vi "test Import Configuration File (Parallel Use).vi"(8 "error in":errorcluster, 11 "TestCase in":refnum<class "Import.lvclass">) -> (0 "error out":errorcluster, 3 "TestCase out":refnum<class "Import.lvclass">)   [LabVIEW 2020, in "Import.lvclass"]
uses:
  Import.lvclass
  <vilib>/addons/_JKI Toolkits/VI Tester/TestCase.llb/TestCase.lvclass
  Import/ARINC 429 Import.lvlib
  niveristand-custom-device-testing-tools/VeriStandTestUtilities/VeriStandTestUtilities.lvlib
  C:/Program Files (x86)/National Instruments/LabVIEW 2020/vi.lib/addons/_JKI Toolkits/VI Tester/TestCase.llb/TestCase.lvclass
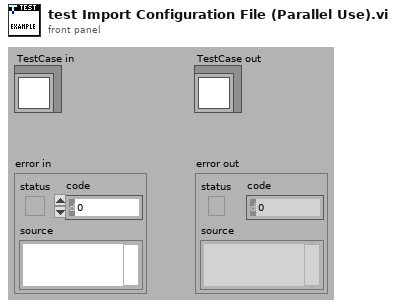
[diagram p1: front panel]
types:
  T1 = typedef "VS Channels Definition for All Labels on Hardware Channel.ctl" = cluster{"hardware channel":i32, "labels":T2[]}
  T2 = typedef "VS Channels Definition for Label.ctl" = cluster{"label (Dec)":u32, "parameters":T3[], "SDI value":u8, "SDI enabled":bool, "transfer type":T7}
  T3 = typedef "VS Channel Definition for Parameter.ctl" = cluster{"name":string, "direction":T4, "default value":dbl, "unit":string, "Parameter":T5}
  T4 = typedef "Direction.ctl" = enum16{"Rx", "Tx"}
  T5 = typedef "Parameter Definition.ctl" = cluster{"start index":i32, "size":i32, "encoding":T6, "signed":bool, "scale multiplier":dbl, "scale offset":dbl}
  T6 = typedef "Encoding and Decoding.lvlib/Encoding.ctl" = enum16{"BNR", "BCD", "Discrete"}
  T7 = typedef "Transfer Type.ctl" = enum16{"Scheduled", "Acyclic", "Block", "Strobe"}
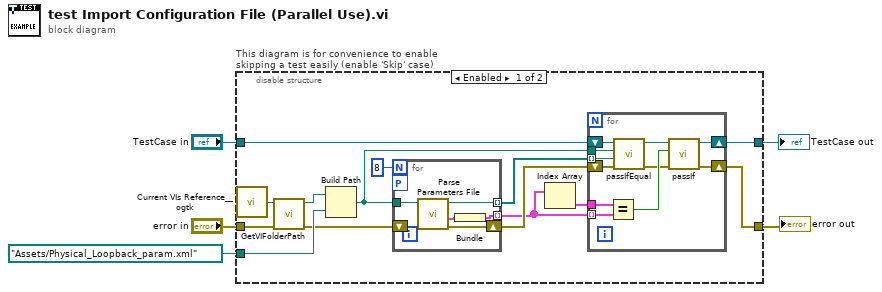
[diagram p0: block diagram]
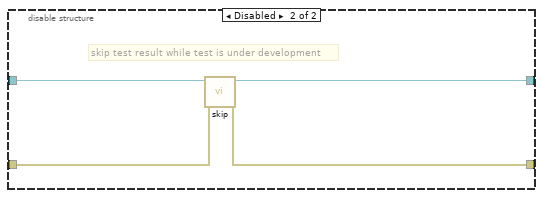
[diagram p2: hidden frame]
diagram:
  n1 = disable-structure "This diagram is for convenience to enable skipping a test easily (enable 'Skip' case)" shown="Enabled" {
    disable-tunnel: "TestCase in" -> [w19 w40]
    disable-tunnel: [w13 w38] -> w2
    disable-tunnel: [w14 w39] -> w4
    disable-tunnel: "error in" -> [w17 w37]
    disable-tunnel: path "Assets/Physical_Loopback_param.xml" ("Absolute or Relative Path") -> [w16 _]
    frame Enabled {
      n2 = call <userlib>:"Current VIs Reference__ogtk.vi"() -> ("Current VI's reference"=w18:refnum<vi>)  [unwired: 5 in]
      n3 = call "GetVIFolderPath.vi"("error in (no error)"=w17, "VI Reference in"=w18) -> ("error out"=w15:errorcluster, "VI Folder Path out"=w12:path)  [unwired: 8 in]
      n4 = Build Path(base path=w12, name or relative path=w16) -> (appended path=w8:path)
      n5 = for {
        N: 8 -> [_]
        tunnel: w8 -> [w35]
        shift-right: [w34] -> w11
        shift-left: w15 -> [w36]
        tunnel: [w32] -> w6 mode=indexing
        tunnel: [w33] -> w9 mode=indexing
        workers-P: _ -> [_]
        n6 = call "Parse Parameters File.vi"("error in"=w36, "path to XML document"=w35) -> ("error out"=w34:errorcluster, "ports"=w31:T1[], "path to XML document out"=w33:path)  [unwired: 7 in]
        n7 = Bundle("ports"=w31) -> (w32:cluster{"ports":T1[]})  [unwired: 1 in]
      }
      n8 = Index Array(array=w6) -> (element=w7:cluster{"ports":T1[]})  [unwired: 1 in]
      n9 = for {
        shift-right: [w28] -> w13
        shift-left: w19 -> [w30]
        shift-right: [w29] -> w14
        shift-left: w11 -> [w26]
        tunnel: w9 -> [w23] mode=indexing
        tunnel: w8 -> [w22]
        tunnel: w7 -> [w21]
        tunnel: w6 -> [w20] mode=indexing
        n10 = Equal?(x=w21, y=w20) -> (x = y?=w27:bool)
        n11 = call-dynamic "passIfEqual.vi"("error in (no error)"=w26, "y"=w23, "x"=w22, "TestCase in"=w30) -> ("error out"=w24:errorcluster, "TestCase out"=w25:refnum<class "Import.lvclass">)  [unwired: 6 in]
        n12 = call-dynamic "passIf.vi"("error in (no error)"=w24, "pass"=w27, "TestCase in"=w25) -> ("error out"=w29:errorcluster, "TestCase out"=w28:refnum<class "Import.lvclass">)  [unwired: 7 in]
      }
    }
    frame Disabled {
      # "skip test result while test is under development"
      n13 = call <vilib>:"skip.vi"("error in (no error)"=w37, "TestCase in"=w40) -> ("error out"=w39:errorcluster, "TestCase out"=w38:refnum<class "Import.lvclass">)  [unwired: 8 in]
    }
  }
  "error out" <- w4
  "TestCase out" <- w2
